vi "Example Callback - Altitude Callback.vi"(4 "Altitude":refnum<user-event>, 5 "Event Data":cluster{"sender":refnum<k24>, "altitude":i32}, 6 "Control Ref":refnum<k24>, 7 "Event Common Data":T1) -> ()   [LabVIEW 2010]
uses:
  C:/tf/play/labview/Tinkerforge.dll
  Tinkerforge.dll
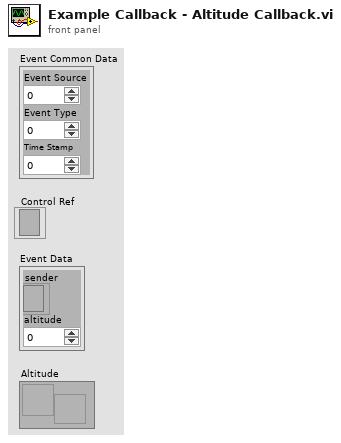
[diagram p1: front panel]
types:
  T1 = cluster{"Event Source":i32, "Event Type":u32, "Time Stamp":u32}
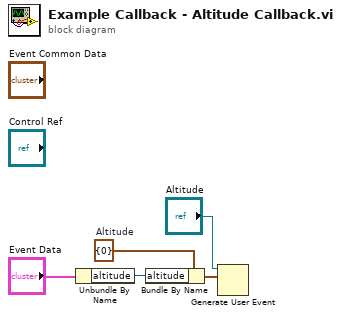
[diagram p0: block diagram]
diagram:
  w4 = cluster{"altitude":i32} {"altitude"=0}  # Altitude
  n1 = Unbundle By Name("Event Data") -> ("altitude"=w3:i32)
  n2 = Bundle By Name(cluster=w4, "altitude"=w3) -> (w2:cluster{"altitude":i32})
  n3 = Generate User Event(user event="Altitude", event data cluster=w2) -> ()  [unwired: 1 in, 2 out]
